vi "Coin Inserted.vi"(8 "error in (no error)":errorcluster, 10 "Coins":bool[](array[boolean]), 11 "Coins in":refnum<class "Coins.lvclass">) -> (0 "error out":errorcluster, 3 "Coins out":refnum<class "Coins.lvclass">)   [LabVIEW 2020, in "Coins.lvlib" / "Coins.lvclass"]
uses:
  Coins.lvclass
  Coins.lvclass/Coins.ctl
  dbfe4258-bbae-4081-b0c7-b73bf81475ff.vi
  <vilib>/Comparison/Equal/Equal Functor/Equal Functor.lvclass
  <vilib>/ActorFramework/Actor/Actor.lvclass
  Controller Messages/Credit and Coin Update Msg/Credit and Coin Update Msg.lvclass
  C:/Program Files (x86)/National Instruments/LabVIEW 2020/vi.lib/ActorFramework/Actor/Actor.lvclass
  D:/Storage/Source Code/Clase AF/ClaseAF/13 Vending Machine/Coins/Coins.lvclass
  D:/Storage/Source Code/Clase AF/ClaseAF/13 Vending Machine/Panel Manager/Panel Manager.lvclass
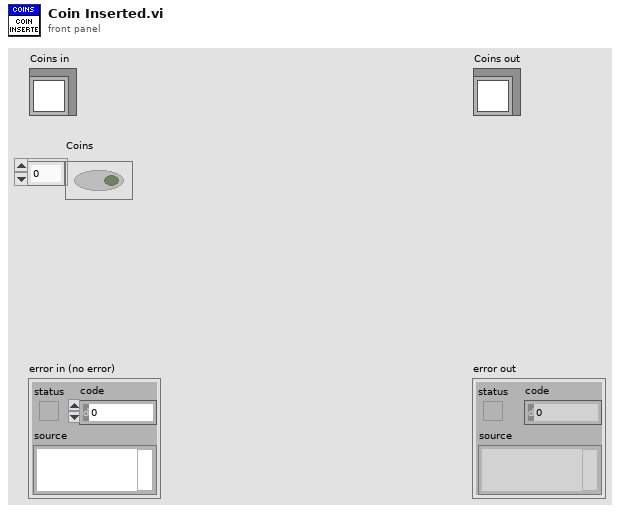
[diagram p1: front panel]
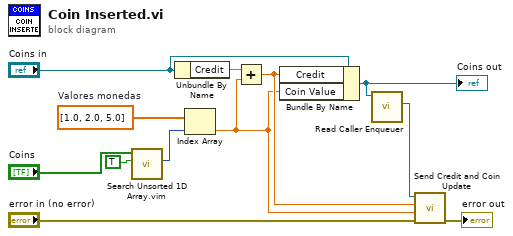
[diagram p0: block diagram]
diagram:
  w10 = dbl[] [1.0, 2.0, 5.0]  # Valores monedas
  n1 = call "Search Unsorted 1D Array.vim"("element"=TRUE, "unsorted 1D array"="Coins") -> ("index of element"=w9:i32)  [unwired: 9 in]
  n2 = Unbundle By Name("Coins in") -> ("Credit"=w7:dbl)
  n3 = Index Array(array=w10, index=w9) -> (element=w3:dbl)
  n4 = Add(x=w7, y=w3) -> (x+y=w4:dbl)
  n5 = Bundle By Name(cluster="Coins in", "Credit"=w4, "Coin Value"=w3) -> (w6:refnum<class "Coins.lvclass">)
  "Coins out" <- w6
  n6 = call <vilib>:"Read Caller Enqueuer.vi"("Actor"=w6) -> ("Caller Enqueuer"=w5:refnum<class "Message Enqueuer.lvclass">)  [unwired: 10 in]
  n7 = call "Send Credit and Coin Update.vi"("error in (no error)"="error in (no error)", "Coin Value"=w3, "Credit"=w4, "Message Enqueuer"=w5) -> ("error out"=→"error out":errorcluster)  [unwired: 6 in, 1 out]
